vi "ux with word.vi"() -> ()   [LabVIEW 2020]
panel:
  in  "Enum":enum16{"Device A", "Device B", "UBD5"}(ring)
  out "Array 3":string[](array[string])
  out "Length in bytes 3":i32
  out "if false  3":string
  out "Result of comparission 3":string
  out "Array 2":string[](array[string])
  out "Length in bytes 2":i32
  out "if false  2":string
  out "Result of comparission 2":string
  out "error out":errorcluster
  out "return value":string
  out "Array":string[](array[string])
  out "Length in bytes":i32
  out "if false":string
  out "Result of comparission":string
  out "Data In":u8[](array[numeric]) format="%.0x"
  out "Batch Length":i32
  out "Actual Bitrate kHz 2":i32=1000
  out "dup Cheetah Handle":i32
  out "Total Shifted Out":i32
  out "Actual Bitrate kHz":i32=1000
  out "error out 2":errorcluster
  in  "Rds per Sec":dbl=2000.0 max=2000000000.0
  out "SDO":u64[](array[numeric]) format="%x"
  in  "SCLK (kHz)":i32=2000 min=0
  out "Cheetah Handle":i32
  out "SDI":u64[](array[numeric]) format="%.0x"
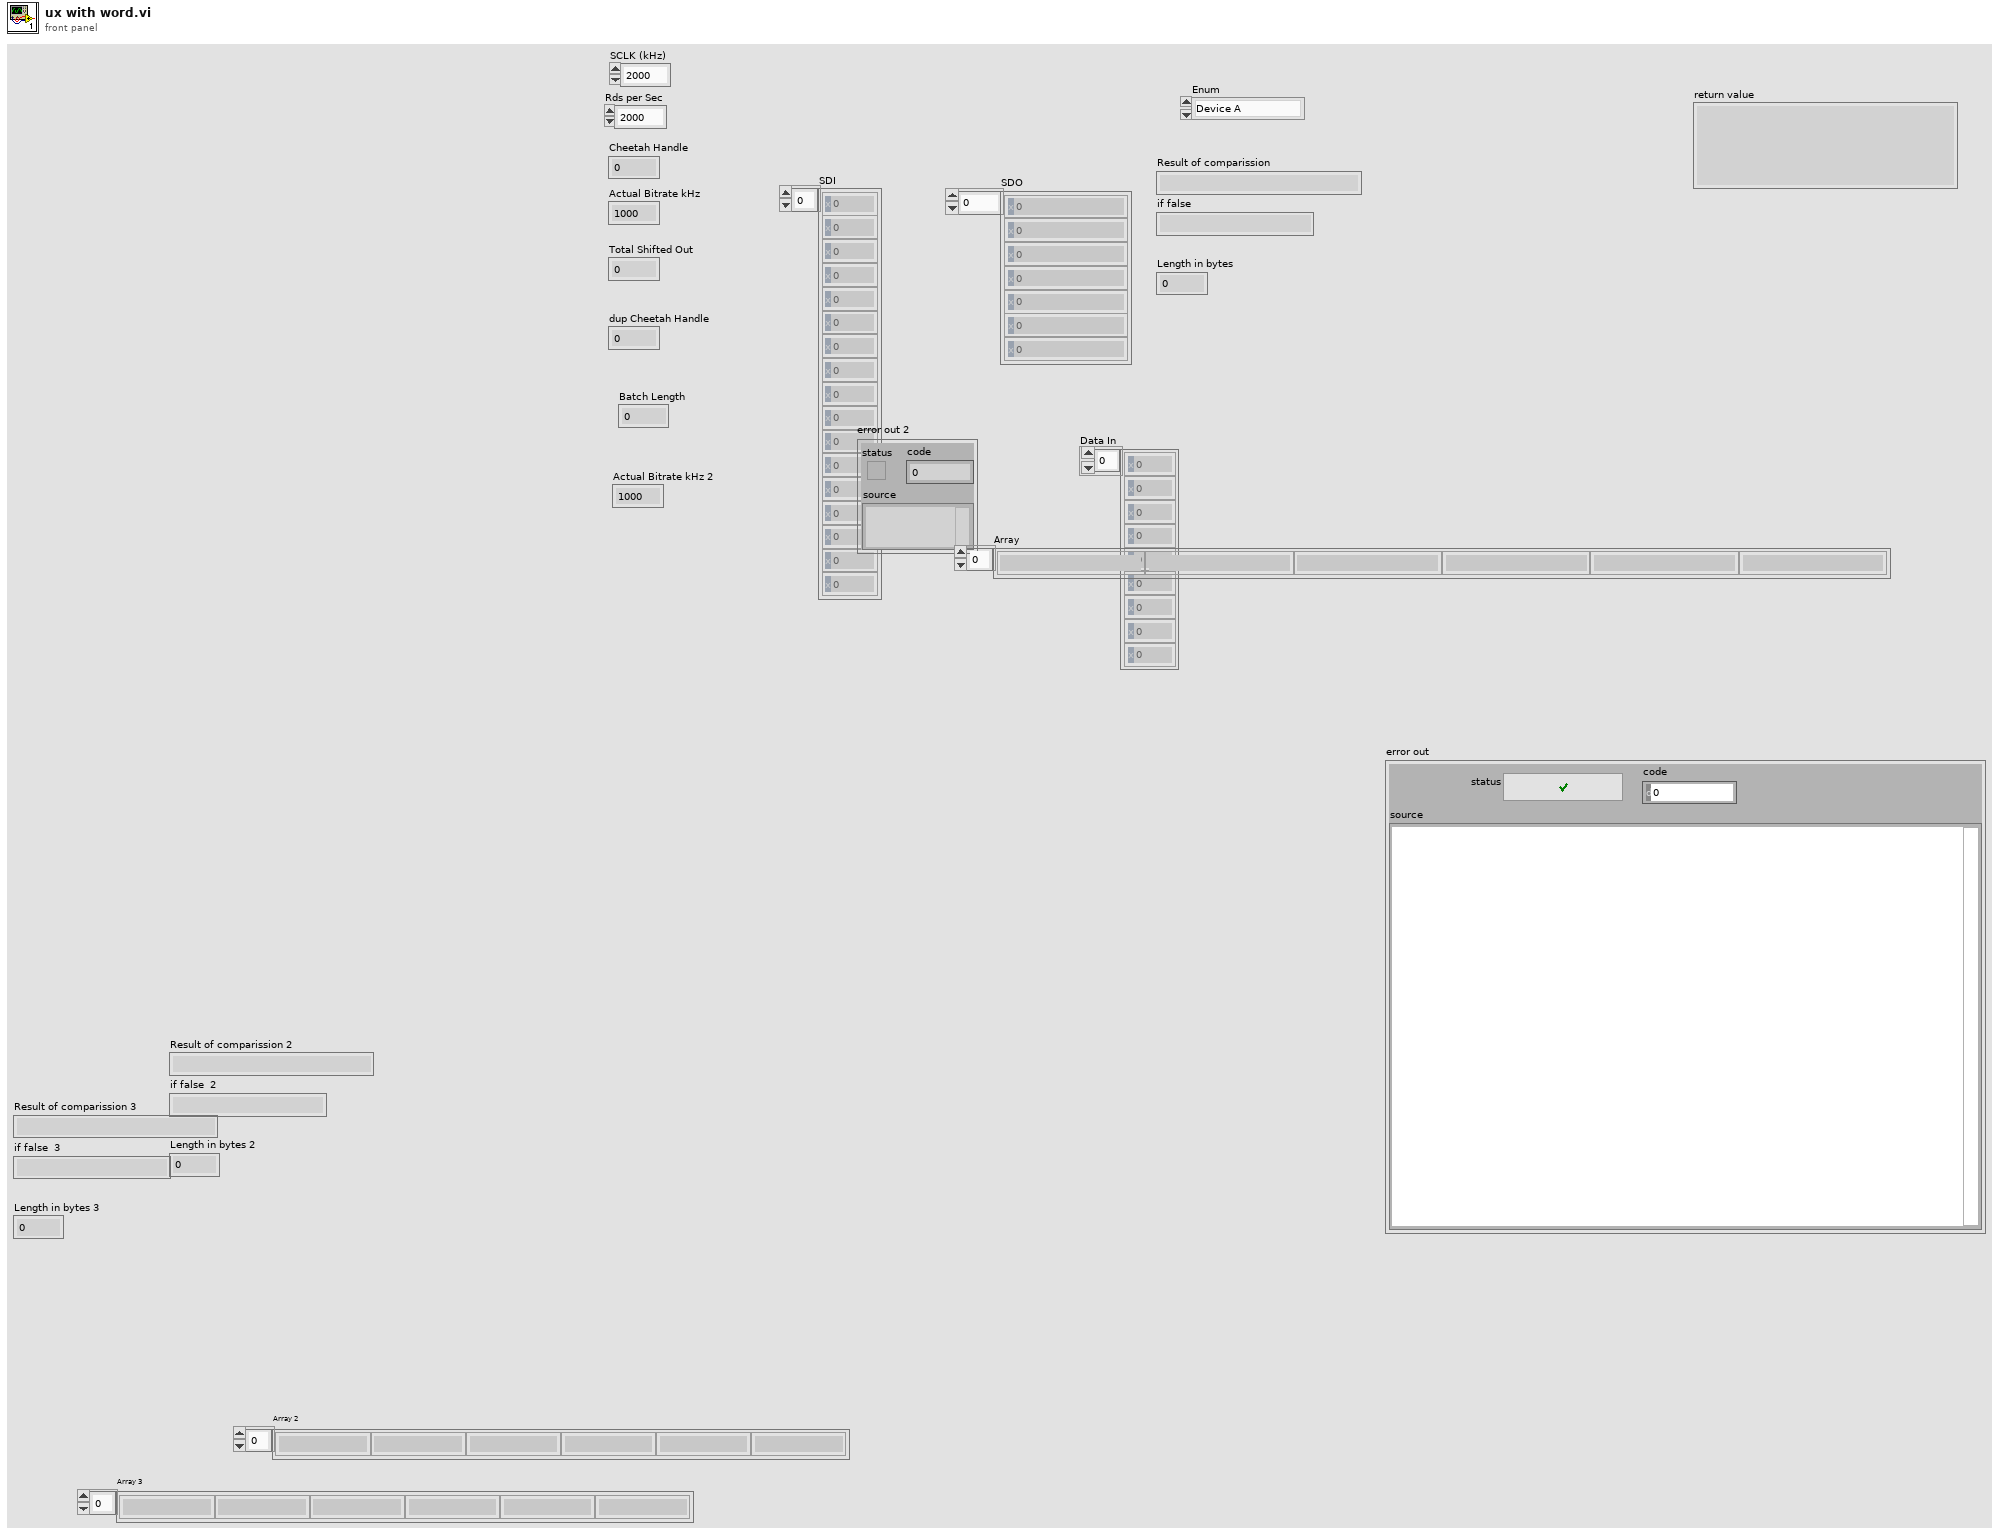
[diagram p1: front panel]
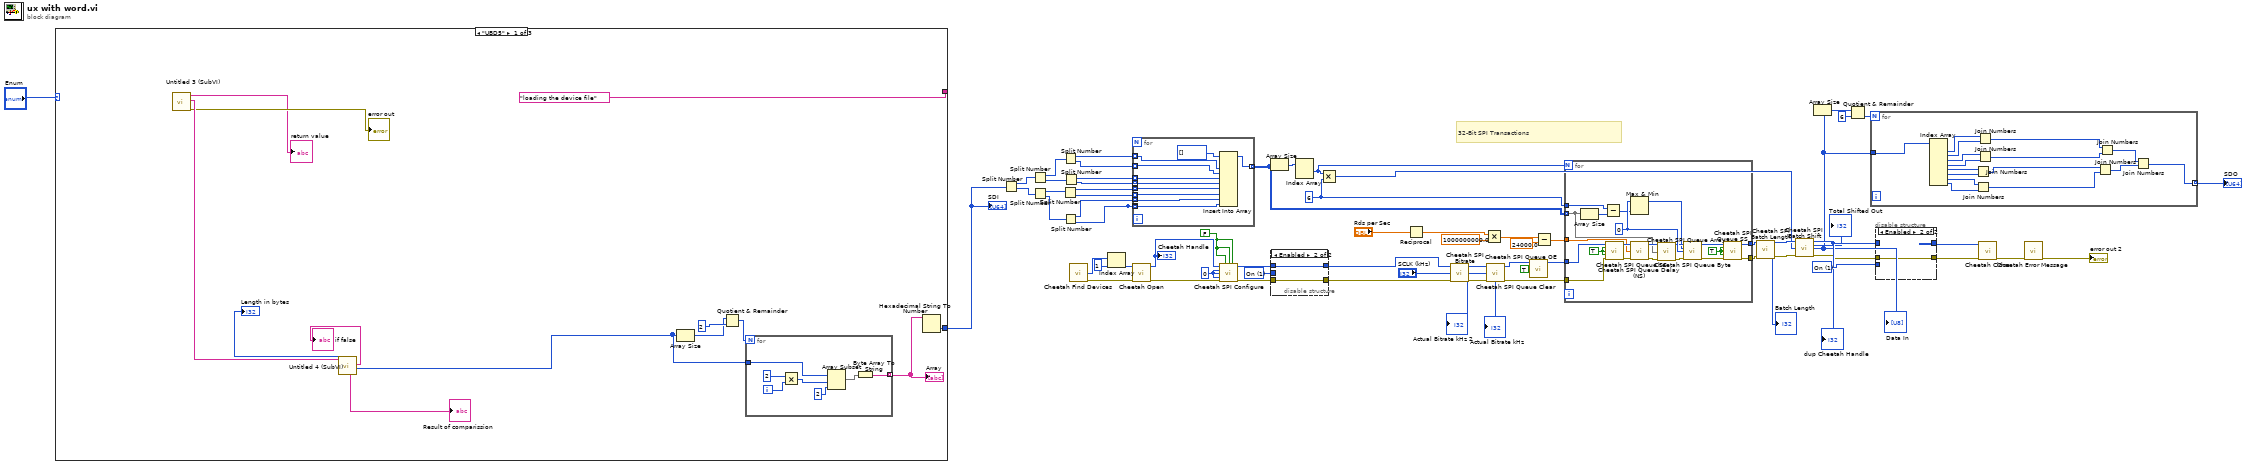
[diagram p0: block diagram]
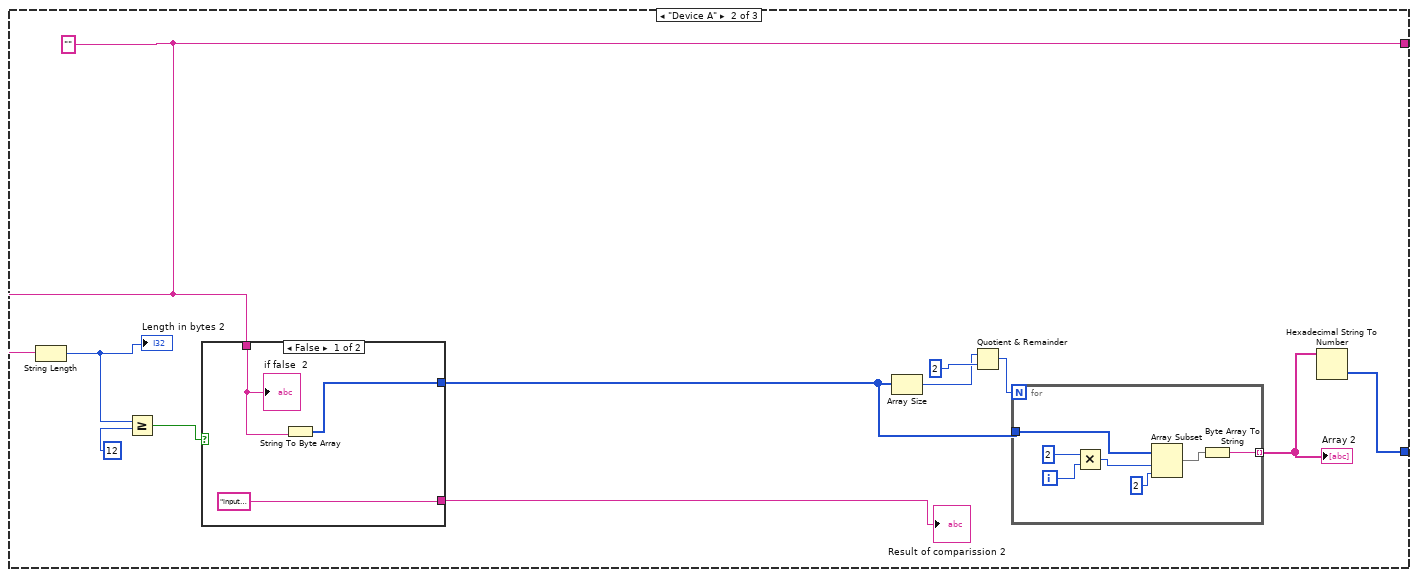
[diagram p2: hidden frame]
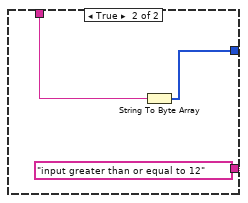
[diagram p3: hidden frame]
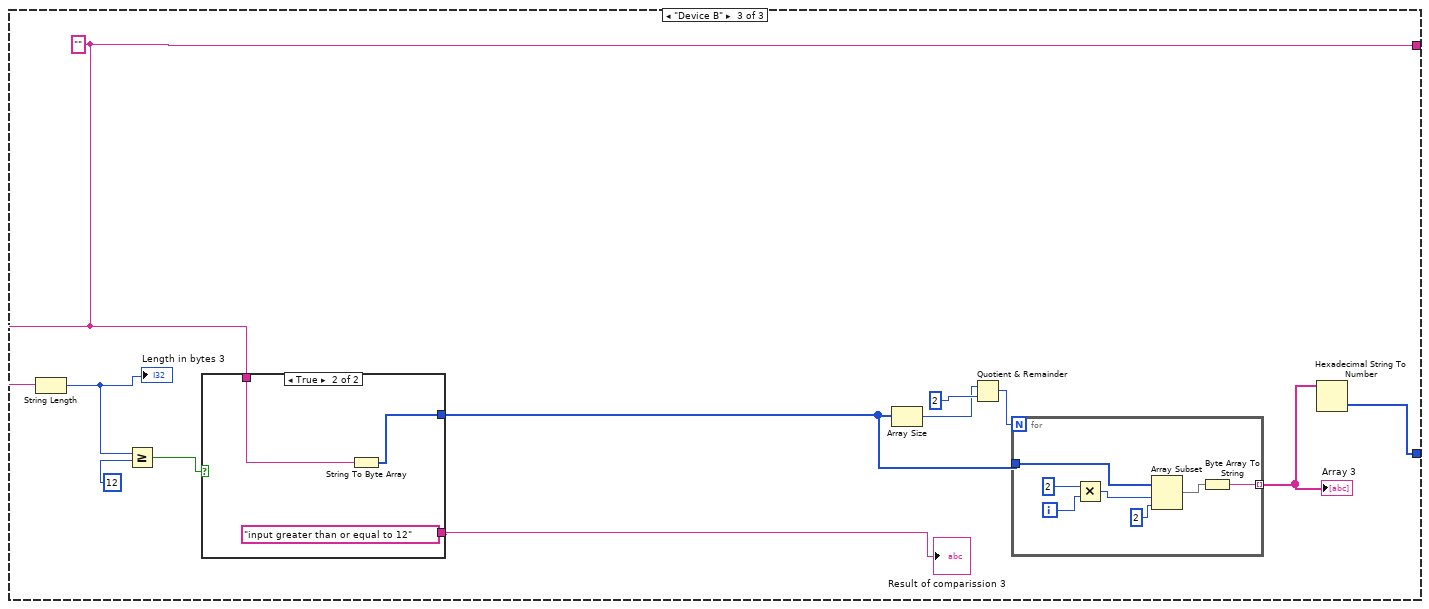
[diagram p4: hidden frame]
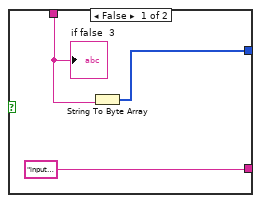
[diagram p5: hidden frame]
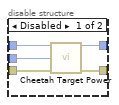
[diagram p6: hidden frame]
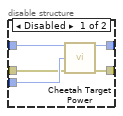
[diagram p7: hidden frame]
diagram:
  w21 = 6 ("y")
  w46 = u16 1 items=["Off", "On", "Query"] ("Requested Configuration (2: Query)")
  w47 = u16 1 items=["Off", "On", "Query"] ("Requested Configuration (2: Query)")
  w62 = FALSE
  w64 = 0
  # "32-Bit SPI Transactions"
  n1 = case shown="\"UBD5\"" "Enum" {
    tunnel: ["loading the device file" w88 w112] -> _
    tunnel: [w71 w87 w111] -> w2
    frame "UBD5" {
      n2 = call "Untitled 3 (SubVI).vi"() -> ("error out"=→"error out":errorcluster, "String"=w72:string, "return value"=→"return value":string)  [unwired: 9 in]
      n3 = call "Untitled 4 (SubVI).vi"("String in"=w72) -> ("unsigned byte array"=w76:u8[], "if false"=→"if false":string, "Length in bytes"=→"Length in bytes":i32, "String out"=→"Result of comparission":string)  [unwired: 7 in]
      n4 = Array Size(array=w76) -> (size(s)=w73:i32)
      n5 = Quotient & Remainder(x=w73, y=2) -> (floor(x/y)=w78:i32)  [unwired: 1 out]
      n6 = for {
        N: w78 -> [_]
        tunnel: w76 -> [w86]
        tunnel: [w83] -> w77 mode=indexing
        i -> [w81]
        n7 = Multiply(x=2 ("y"), y=w81) -> (x*y=w85:i32)
        n8 = Array Subset(array=w86, index=w85, length=2) -> (w82:u8[])
        n9 = Byte Array To String(unsigned byte array=w82) -> (string=w83:string)
      }
      "Array" <- w77
      n10 = Hexadecimal String To Number(string=w77) -> (number=w71:u32[])  [unwired: 2 in, 1 out]
    }
    frame "Device A" {
      w88 = ""
      n11 = String Length(string=w88) -> (length=w91:i32)
      "Length in bytes 2" <- w91
      n12 = Greater Or Equal?(x=w91, y=12) -> (x >= y?=w94:bool)
      n13 = case shown="False" w94 {
        tunnel: [w98 w103] -> w93
        tunnel: w88 -> [w99 w102]
        tunnel: ["input less than 12" "input greater than or equal to 12"] -> w92
        frame False {
          n14 = String To Byte Array(string=w99) -> (unsigned byte array=w98:u8[])
          "if false  2" <- w99
        }
        frame True {
          n15 = String To Byte Array(string=w102) -> (unsigned byte array=w103:u8[])
        }
      }
      "Result of comparission 2" <- w92
      n16 = Array Size(array=w93) -> (size(s)=w89:i32)
      n17 = Quotient & Remainder(x=w89, y=2) -> (floor(x/y)=w97:i32)  [unwired: 1 out]
      n18 = for {
        N: w97 -> [_]
        tunnel: w93 -> [w110]
        tunnel: [w107] -> w96 mode=indexing
        i -> [w105]
        n19 = Multiply(x=2 ("y"), y=w105) -> (x*y=w109:i32)
        n20 = Array Subset(array=w110, index=w109, length=2) -> (w106:u8[])
        n21 = Byte Array To String(unsigned byte array=w106) -> (string=w107:string)
      }
      "Array 2" <- w96
      n22 = Hexadecimal String To Number(string=w96) -> (number=w87:u32[])  [unwired: 2 in, 1 out]
    }
    frame "Device B" {
      w112 = ""
      n23 = String Length(string=w112) -> (length=w115:i32)
      "Length in bytes 3" <- w115
      n24 = Greater Or Equal?(x=w115, y=12) -> (x >= y?=w118:bool)
      n25 = case shown="True" w118 {
        tunnel: [w122 w127] -> w117
        tunnel: w112 -> [w123 w126]
        tunnel: ["input less than 12" "input greater than or equal to 12"] -> w116
        frame False {
          n26 = String To Byte Array(string=w123) -> (unsigned byte array=w122:u8[])
          "if false  3" <- w123
        }
        frame True {
          n27 = String To Byte Array(string=w126) -> (unsigned byte array=w127:u8[])
        }
      }
      "Result of comparission 3" <- w116
      n28 = Array Size(array=w117) -> (size(s)=w113:i32)
      n29 = Quotient & Remainder(x=w113, y=2) -> (floor(x/y)=w121:i32)  [unwired: 1 out]
      n30 = for {
        N: w121 -> [_]
        tunnel: w117 -> [w134]
        tunnel: [w131] -> w120 mode=indexing
        i -> [w129]
        n31 = Multiply(x=2 ("y"), y=w129) -> (x*y=w133:i32)
        n32 = Array Subset(array=w134, index=w133, length=2) -> (w130:u8[])
        n33 = Byte Array To String(unsigned byte array=w130) -> (string=w131:string)
      }
      "Array 3" <- w120
      n34 = Hexadecimal String To Number(string=w120) -> (number=w111:u32[])  [unwired: 2 in, 1 out]
    }
  }
  "SDI" <- w2
  n35 = Split Number(x=w2) -> (hi(x)=w32:u16[], lo(x)=w31:u16[])
  n36 = Split Number(x=w32) -> (hi(x)=w9:u8[], lo(x)=w8:u8[])
  n37 = Split Number(x=w31) -> (hi(x)=w11:u8[], lo(x)=w10:u8[])
  n38 = Split Number(x=w11) -> (hi(x)=w15:u8[], lo(x)=w14:u8[])
  n39 = Split Number(x=w9) -> (hi(x)=w7:u8[], lo(x)=w6:u8[])
  n40 = Split Number(x=w10) -> (hi(x)=w13:u8[], lo(x)=w12:u8[])
  n41 = Split Number(x=w8) -> (hi(x)=w5:u8[], lo(x)=w4:u8[])
  n42 = call <instrlib>:"Cheetah Find Devices.vi"() -> ("Ports"=w65:u16[], "error out"=w61:errorcluster)  [unwired: 13 in, 1 out]
  n43 = Index Array(array=w65, index=1) -> (element=w53:u16)
  n44 = for {
    tunnel: w15 -> [w144] mode=indexing
    tunnel: [w143] -> w30 mode=indexing
    tunnel: w13 -> [w141] mode=indexing
    tunnel: w12 -> [_] mode=indexing
    tunnel: w12 -> [w140] mode=indexing
    tunnel: w14 -> [w139] mode=indexing
    tunnel: w7 -> [w138] mode=indexing
    tunnel: w6 -> [w137] mode=indexing
    tunnel: w5 -> [w136] mode=indexing
    tunnel: w4 -> [w135] mode=indexing
    n45 = Insert Into Array(array=u8[] [], new element #1=w138, new element #2=w137, new element #3=w136, new element #4=w135, new element #5=w144, new element #6=w139, new element #7=w141, new element #8=w140) -> (w143:u8[])  [unwired: 1 in]
  }
  n46 = call <instrlib>:"Cheetah Open.vi"("Port Number (0)"=w53, "error in (no error)"=w61) -> ("Cheetah Handle"=w58:i32, "error out"=w60:errorcluster)  [unwired: 12 in]
  "Cheetah Handle" <- w58
  n47 = call <instrlib>:"Cheetah SPI Configure.vi"("Cheetah Handle"=w58, "SS0 Active High? (False)"=w62, "SS1 Active High? (False)"=w62, "SS2 Active High? (False)"=w62, "Polarity (0: Rising/Falling)"=w64, "Phase (0: Sample/Setup)"=w64, "Bitorder (0: MSB)"=w64, "error in (no error)"=w60) -> ("dup Cheetah Handle"=w57:i32, "error out"=w59:errorcluster)  [unwired: 6 in]
  n48 = Array Size(array=w30) -> (size(s)=w45:i32[])
  n49 = disable-structure shown="Enabled" {
    disable-tunnel: w59 -> [w149 w150]
    disable-tunnel: w57 -> [w148 w151]
    disable-tunnel: [w147 w150] -> w56
    disable-tunnel: [w146 w151] -> w54
    disable-tunnel: w46 -> [w145 _]
    frame Disabled {
      n50 = call <instrlib>:"Cheetah Target Power.vi"("Cheetah Handle"=w148, "Requested Configuration (2: Query)"=w145, "error in (no error)"=w149) -> ("dup Cheetah Handle"=w146:i32, "error out"=w147:errorcluster)  [unwired: 10 in, 1 out]
    }
    frame Enabled {
    }
  }
  n51 = Index Array(array=w45) -> (element #1=w17:i32)  [unwired: 2 in, 1 out]
  n52 = Multiply(x=w17, y=w21) -> (x*y=w16:i32)
  n53 = Reciprocal(x="Rds per Sec") -> (1/x=w23:dbl)
  n54 = call <instrlib>:"Cheetah SPI Bitrate.vi"("Cheetah Handle"=w54, "Requested Bitrate kHz (1000)"="SCLK (kHz)", "error in (no error)"=w56) -> ("dup Cheetah Handle"=w52:i32, "Actual Bitrate kHz"=→"Actual Bitrate kHz" →"Actual Bitrate kHz 2":i32, "error out"=w51:errorcluster)  [unwired: 10 in]
  n55 = Multiply(x=w23, y=1000000000.0) -> (x*y=w26:dbl)
  n56 = call <instrlib>:"Cheetah SPI Queue Clear.vi"("Cheetah Handle"=w52, "error in (no error)"=w51) -> ("dup Cheetah Handle"=w44:i32, "error out"=w63:errorcluster)  [unwired: 12 in]
  n57 = call <instrlib>:"Cheetah SPI Queue OE.vi"("Cheetah Handle"=w44, "Output Enable (on)"=TRUE) -> ("dup Cheetah Handle"=w43:i32)  [unwired: 12 in, 1 out]
  n58 = Subtract(x=w26, y=24000.0) -> (x-y=w24:dbl)
  n59 = for {
    N: w17 -> [_]
    tunnel: w63 -> [w158]
    tunnel: w43 -> [w159]
    tunnel: w30 -> [w160] mode=indexing
    tunnel: [w157] -> w41
    tunnel: [w156] -> w40
    tunnel: w24 -> [w153]
    tunnel: w21 -> [w154]
    w164 = TRUE
    w167 = 0
    w155 = TRUE
    n60 = Array Size(array=w160) -> (size(s)=w161:i32)
    n61 = Subtract(x=w154, y=w161) -> (x-y=w165:i32)
    n62 = call <instrlib>:"Cheetah SPI Queue SS.vi"("Cheetah Handle"=w159, "SS0 Assert? (True)"=w155, "SS1 Assert? (True)"=w155, "SS2 Assert? (True)"=w155, "error in (no error)"=w158) -> ("dup Cheetah Handle"=w172:i32, "error out"=w171:errorcluster)  [unwired: 9 in]
    n63 = Max & Min(x=w167, y=w165) -> (max(x,y)=w152:i32)  [unwired: 1 out]
    n64 = call <instrlib>:"Cheetah SPI Queue Delay (NS).vi"("Cheetah Handle"=w172, "Delay NS (1000)"=w153, "error in (no error)"=w171) -> ("dup Cheetah Handle"=w170:i32, "error out"=w169:errorcluster)  [unwired: 10 in, 1 out]
    n65 = call <instrlib>:"Cheetah SPI Queue Array.vi"("Cheetah Handle"=w170, "Data Out (none)"=w160, "error in (no error)"=w169) -> ("dup Cheetah Handle"=w166:i32, "error out"=w168:errorcluster)  [unwired: 11 in]
    n66 = call <instrlib>:"Cheetah SPI Queue Byte.vi"("Cheetah Handle"=w166, "Byte Count (1)"=w152, "Byte Value (0x00)"=w167, "error in (no error)"=w168) -> ("dup Cheetah Handle"=w163:i32, "error out"=w162:errorcluster)  [unwired: 10 in]
    n67 = call <instrlib>:"Cheetah SPI Queue SS.vi"("Cheetah Handle"=w163, "SS0 Assert? (True)"=w164, "SS1 Assert? (True)"=w164, "SS2 Assert? (True)"=w164, "error in (no error)"=w162) -> ("dup Cheetah Handle"=w156:i32, "error out"=w157:errorcluster)  [unwired: 9 in]
  }
  n68 = call <instrlib>:"Cheetah SPI Batch Length.vi"("Cheetah Handle"=w40, "error in (no error)"=w41) -> ("dup Cheetah Handle"=w39:i32, "Batch Length"=→"Batch Length":i32, "error out"=w38:errorcluster)  [unwired: 11 in]
  n69 = call <instrlib>:"Cheetah SPI Batch Shift.vi"("Cheetah Handle"=w39, "Max Bytes to Retrieve (256)"=w16, "error in (no error)"=w38) -> ("dup Cheetah Handle"=w37:i32, "Total Shifted Out"=→"Total Shifted Out":i32, "Data In"=w18:u8[], "error out"=w29:errorcluster)  [unwired: 9 in]
  "dup Cheetah Handle" <- w37
  "Data In" <- w18
  n70 = Array Size(array=w18) -> (size(s)=w36:i32)
  n71 = Quotient & Remainder(x=w36, y=6) -> (floor(x/y)=w34:i32)  [unwired: 1 out]
  n72 = for {
    N: w34 -> [_]
    tunnel: w18 -> [w187]
    tunnel: [w186] -> w33 mode=indexing
    n73 = Index Array(array=w187) -> (element #1=w176:u8, element #2=w175:u8, element #3=w174:u8, element #4=w173:u8, element #5=w185:u8, element #6=w184:u8, element #7=w183:u8, element #8=w182:u8)  [unwired: 8 in]
    n74 = Join Numbers(hi=w185, lo=w184) -> ((hi.lo)=w181:u16)
    n75 = Join Numbers(hi=w183, lo=w182) -> ((hi.lo)=w180:u16)
    n76 = Join Numbers(hi=w176, lo=w175) -> ((hi.lo)=w179:u16)
    n77 = Join Numbers(hi=w174, lo=w173) -> ((hi.lo)=w178:u16)
    n78 = Join Numbers(hi=w181, lo=w180) -> ((hi.lo)=w188:u32)
    n79 = Join Numbers(hi=w179, lo=w178) -> ((hi.lo)=w177:u32)
    n80 = Join Numbers(hi=w177, lo=w188) -> ((hi.lo)=w186:u64)
  }
  "SDO" <- w33
  n81 = disable-structure shown="Enabled" {
    disable-tunnel: [w193 _] -> w50
    disable-tunnel: [w192 w194] -> w49
    disable-tunnel: w47 -> [w191 _]
    disable-tunnel: w37 -> [w190 _]
    disable-tunnel: w29 -> [w189 w194]
    frame Disabled {
      n82 = call <instrlib>:"Cheetah Target Power.vi"("Cheetah Handle"=w190, "Requested Configuration (2: Query)"=w191, "error in (no error)"=w189) -> ("dup Cheetah Handle"=w193:i32, "error out"=w192:errorcluster)  [unwired: 10 in, 1 out]
    }
    frame Enabled {
    }
  }
  n83 = call <instrlib>:"Cheetah Close.vi"("Cheetah Handle"=w50, "error in (no error)"=w49) -> ("error out"=w48:errorcluster)  [unwired: 12 in, 1 out]
  n84 = call <instrlib>:"Cheetah Error Message.vi"("error in (no error)"=w48) -> ("error out"=→"error out 2":errorcluster)  [unwired: 10 in, 4 out]
